vi "___save_1d_text_with_header.vi"(6 "ヘッダー":string, 7 "プロンプト":string, 8 "配列":string[](array[string]), 10 "file_name":string, 11 "パス":path) -> (3 "出力パス":path)   [LabVIEW 2017]
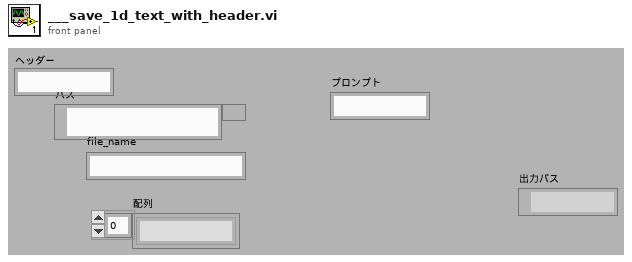
[diagram p1: front panel]
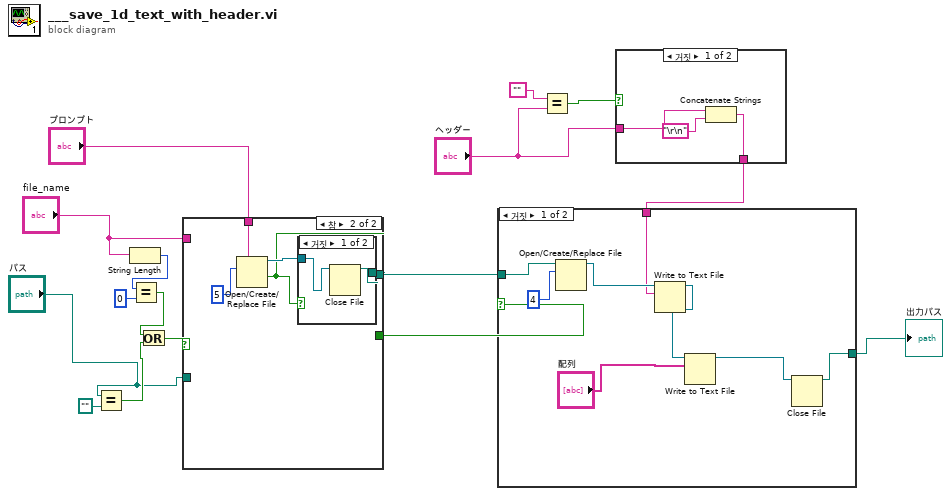
[diagram p0: block diagram]
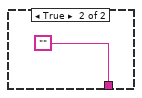
[diagram p2: hidden frame]
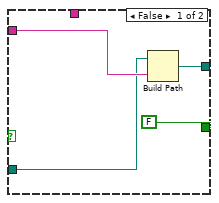
[diagram p4: hidden frame]
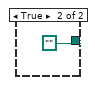
[diagram p5: hidden frame]
diagram:
  n1 = Equal?(x="パス", y=path "") -> (x = y?=w2:bool)
  n2 = String Length(string="file_name") -> (length=w16:i32)
  n3 = Equal?(x=w16, y=0) -> (x = y?=w3:bool)
  n4 = Or(x=w3, y=w2) -> (x .or. y?=w4:bool)
  n5 = case shown="참" w4 {
    tunnel: "file_name" -> [w20 _]
    tunnel: [w19 w23] -> w12
    tunnel: [FALSE w22] -> w13
    tunnel: "プロンプト" -> [_ w21]
    tunnel: "パス" -> [w17 _]
    frame False {
      n6 = Build Path(base path=w17, name or relative path=w20) -> (appended path=w19:path)
    }
    frame True {
      n7 = Open/Create/Replace File(prompt=w21, operation (0:open)=5) -> (refnum out=w24:refnum<file>, cancelled=w22:bool)  [unwired: 4 in, 1 out]
      n8 = case shown="거짓" w22 {
        tunnel: w24 -> [w27 _]
        tunnel: [w26 path ""] -> w23
        frame False {
          n9 = Close File(refnum=w27) -> (path=w26:path)  [unwired: 1 in, 1 out]
        }
        frame True {
        }
      }
    }
  }
  n10 = Equal?(x="", y="ヘッダー") -> (x = y?=w8:bool)
  n11 = case shown="거짓" w8 {
    tunnel: "ヘッダー" -> [w30 _]
    tunnel: [w29 ""] -> w6
    frame False {
      n12 = Concatenate Strings(w30, "\r\n") -> (w29:string)
    }
    frame True {
    }
  }
  n13 = case shown="거짓" w13 {
    tunnel: w12 -> [w40 w41]
    tunnel: w6 -> [w37 _]
    tunnel: [w34 w41] -> w10
    frame False {
      n14 = Open/Create/Replace File(file path (use dialog)=w40, operation (0:open)=4) -> (refnum out=w38:refnum<file>)  [unwired: 4 in, 2 out]
      n15 = Write to Text File(file (use dialog)=w38, text=w37) -> (refnum out=w36:refnum<file>)  [unwired: 2 in, 2 out]
      n16 = Write to Text File(file (use dialog)=w36, text="配列") -> (refnum out=w35:refnum<file>)  [unwired: 2 in, 2 out]
      n17 = Close File(refnum=w35) -> (path=w34:path)  [unwired: 1 in, 1 out]
    }
    frame True {
    }
  }
  "出力パス" <- w10
